vi "q3 full adder.vi"() -> ()   [LabVIEW 2025]
panel:
  out "CARRY":bool
  out "SUM":bool
  in  "CIN":bool
  in  "B":bool
  in  "A":bool
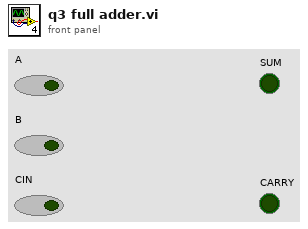
[diagram p1: front panel]
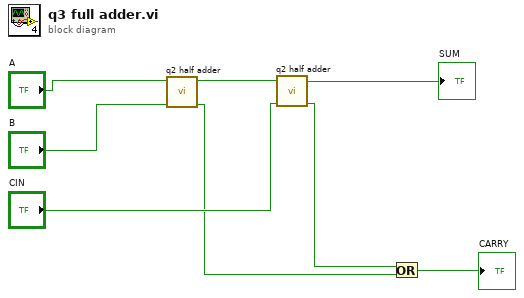
[diagram p0: block diagram]
diagram:
  n1 = call "q2 half adder.vi"("B"="B", "A"="A") -> ("CARRY"=w3:bool, "SUM"=w5:bool)  [unwired: 8 in]
  n2 = call "q2 half adder.vi"("B"="CIN", "A"=w5) -> ("CARRY"=w4:bool, "SUM"=→"SUM":bool)  [unwired: 8 in]
  n3 = Or(x=w4, y=w3) -> (x .or. y?=→"CARRY":bool)
